vi "FlatToRichnixnet_grpc_ReadStateRequest.vi"(5 "OutputClusterType":T1, 11 "InputCluster":T3) -> (3 "OutputCluster":T1)   [LabVIEW 2025, in "grpc-xnet_client.lvlib"]
uses:
  nixnet_grpc_ReadStateRequest_Flat.ctl
  nidevice_grpc_Session_Flat.ctl
  nixnet_grpc_ReadState.ctl
  nixnet_grpc_ReadStateRequest.ctl
  nixnet_grpc_ReadStateRequest_state_id_enum/nixnet_grpc_ReadStateRequest_state_id_enum.lvclass
  nidevice_grpc_Session.ctl
  grpc-xnet_client.lvlib
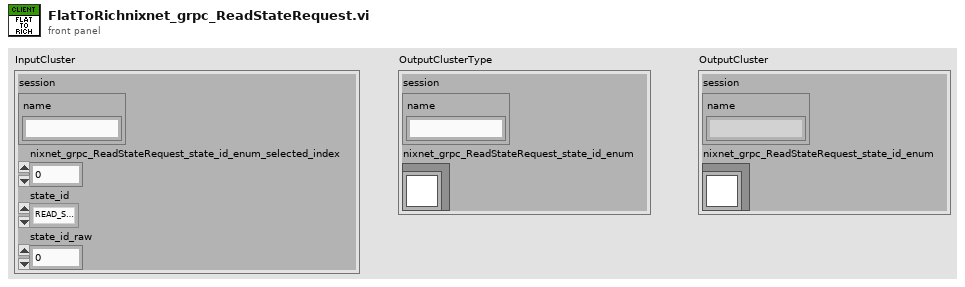
[diagram p1: front panel]
types:
  T1 = typedef "grpc-xnet_client.lvlib/nixnet_grpc_ReadStateRequest.ctl" = cluster{"session":T2, "nixnet_grpc_ReadStateRequest_state_id_enum":refnum<class "nixnet_grpc_ReadStateRequest_state_id_enum.lvclass">}
  T2 = typedef "grpc-xnet_client.lvlib/nidevice_grpc_Session.ctl" = cluster{"name":string}
  T3 = typedef "grpc-xnet_client.lvlib/nixnet_grpc_ReadStateRequest_Flat.ctl" = cluster{"session":T4, "nixnet_grpc_ReadStateRequest_state_id_enum_selected_index":i32, "state_id":T5, "state_id_raw":u32}
  T4 = typedef "grpc-xnet_client.lvlib/nidevice_grpc_Session_Flat.ctl" = cluster{"name":string}
  T5 = typedef "grpc-xnet_client.lvlib/nixnet_grpc_ReadState.ctl" = enum32{"READ_STATE_UNSPECIFIED", "READ_STATE_TIME_CURRENT", "READ_STATE_TIME_COMMUNICATING", "READ_STATE_TIME_START", "READ_STATE_SESSION_INFO", "READ_STATE_TIME_CURRENT_2", "READ_STATE_TIME_COMMUNICATING_2", "READ_STATE_TIME_START_2", "READ_STATE_CAN_COMM", "READ_STATE_FLEX_RAY_COMM", "READ_STATE_FLEX_RAY_STATS", "READ_STATE_LIN_COMM", "READ_STATE_J1939_COMM"}
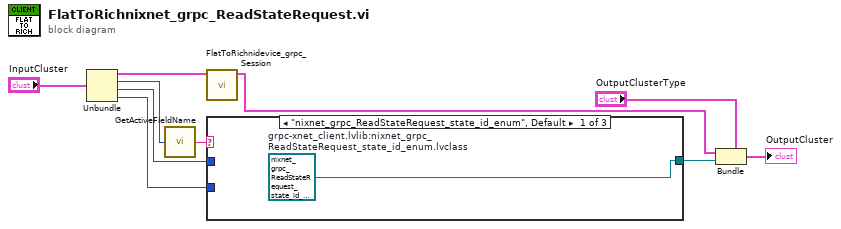
[diagram p0: block diagram]
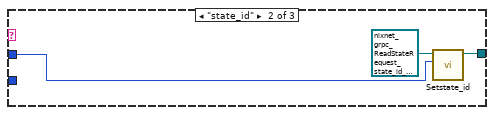
[diagram p2: hidden frame]
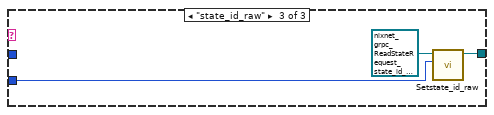
[diagram p3: hidden frame]
diagram:
  n1 = Unbundle "Unbundle"("InputCluster") -> ("session"=w7:T4, "nixnet_grpc_ReadStateRequest_state_id_enum_selected_index"=w5:i32, "state_id"=w2:T5, "state_id_raw"=w1:u32)
  n2 = call "GetActiveFieldName.vi"("protobuf index"=w5) -> ("oneof field name"=w4:string)
  n3 = call "FlatToRichnidevice_grpc_Session.vi"("InputCluster"=w7) -> ("OutputCluster"=w6:T2)  [unwired: 10 in]
  n4 = case "nixnet_grpc_ReadStateRequest_state_id_enum" shown="\"nixnet_grpc_ReadStateRequest_state_id_enum\", Default" w4 {
    tunnel: [w11 w13 w16] -> w3
    tunnel: w2 -> [_ w14 _]
    tunnel: w1 -> [_ _ w17]
    frame "nixnet_grpc_ReadStateRequest_state_id_enum", Default {
      w11 = refnum<class "nixnet_grpc_ReadStateRequest_state_id_enum.lvclass"> refnum  # grpc-xnet_client.lvlib:nixnet_grpc_ReadStateRequest_state_id_enum.lvclass
    }
    frame "state_id" {
      n5 = call "Setstate_id.vi"("Set_Val"=w14, "OneOfTemplate in"=refnum<class "nixnet_grpc_ReadStateRequest_state_id_enum.lvclass"> refnum) -> ("OneOfTemplate out"=w13:refnum<class "nixnet_grpc_ReadStateRequest_state_id_enum.lvclass">)  [unwired: 8 in, 1 out]
    }
    frame "state_id_raw" {
      n6 = call "Setstate_id_raw.vi"("Set_Val"=w17, "OneOfTemplate in"=refnum<class "nixnet_grpc_ReadStateRequest_state_id_enum.lvclass"> refnum) -> ("OneOfTemplate out"=w16:refnum<class "nixnet_grpc_ReadStateRequest_state_id_enum.lvclass">)  [unwired: 8 in, 1 out]
    }
  }
  n7 = Bundle "Bundle"(cluster="OutputClusterType", "session"=w6, "nixnet_grpc_ReadStateRequest_state_id_enum"=w3) -> (→"OutputCluster":T1)
